vi "control.vi"() -> ()   [LabVIEW 2011]
uses:
  Controls/States.ctl
  <vilib>/Instr/_visa.llb/VISA Configure Serial Port (Instr).vi
panel:
  out "read buffer":string
  in  "Vertical Pointer Slide":dbl(slide) scale=0.0..100.0
  in  "Stop Button":bool
  in  "VISA resource name":refnum<visa-resource-name>
  in  "Stop Motion":bool caption="Stop"
  in  "Right":bool
  in  "Left":bool
  in  "Forward":bool
  in  "Back":bool
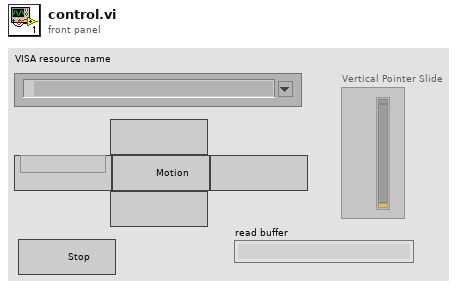
[diagram p1: front panel]
types:
  T1 = typedef "States.ctl" = enum16{"Init", "Idle", "AckCommand", "CheckError", "Shutdown"}
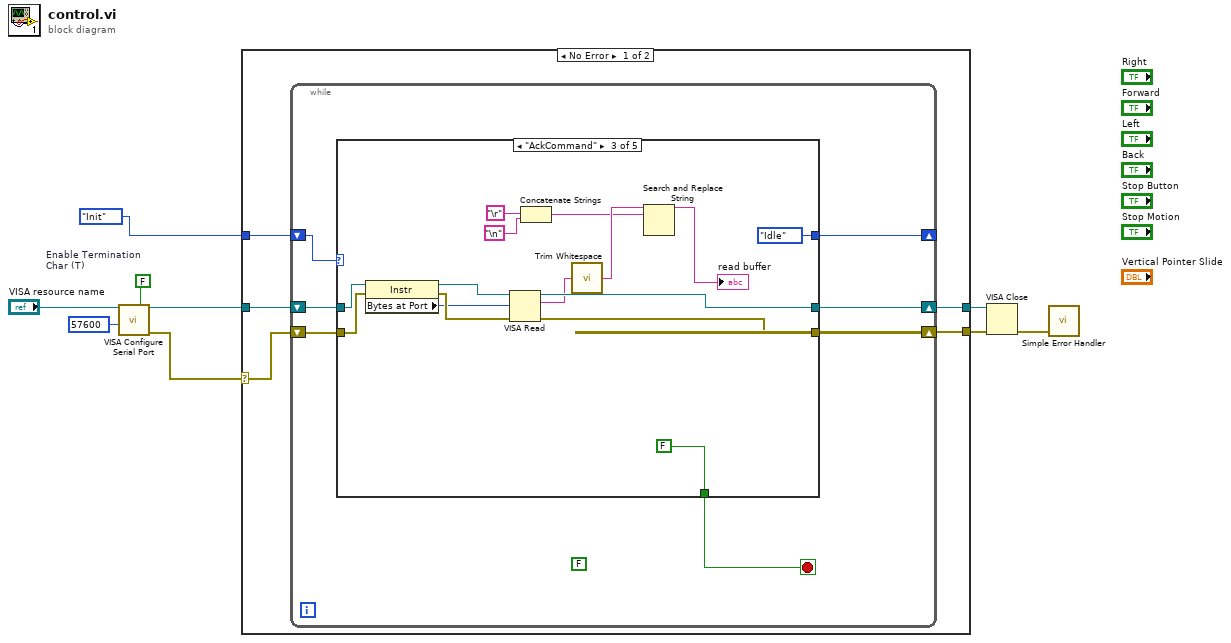
[diagram p0: block diagram]
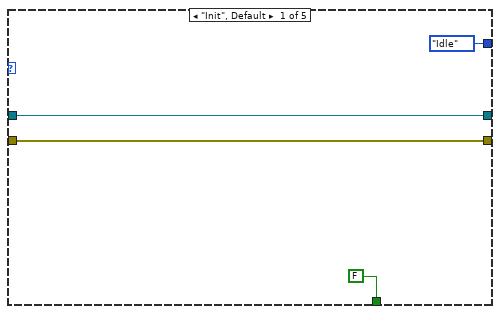
[diagram p2: hidden frame]
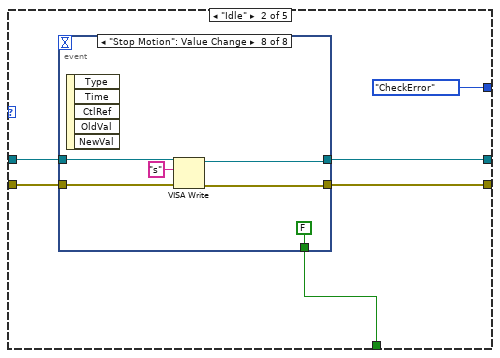
[diagram p3: hidden frame]
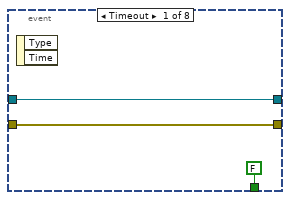
[diagram p4: hidden frame]
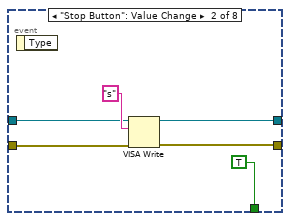
[diagram p5: hidden frame]
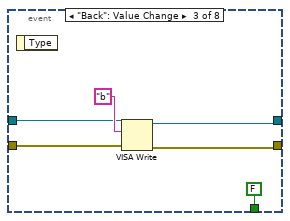
[diagram p6: hidden frame]
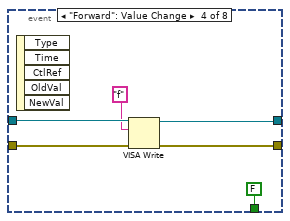
[diagram p7: hidden frame]
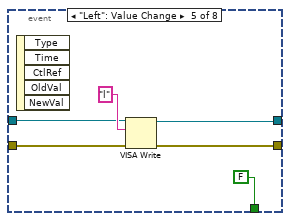
[diagram p8: hidden frame]
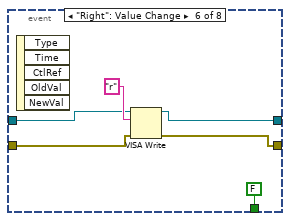
[diagram p9: hidden frame]
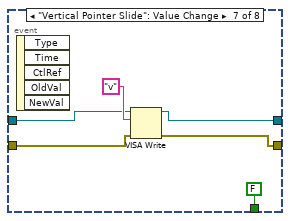
[diagram p10: hidden frame]
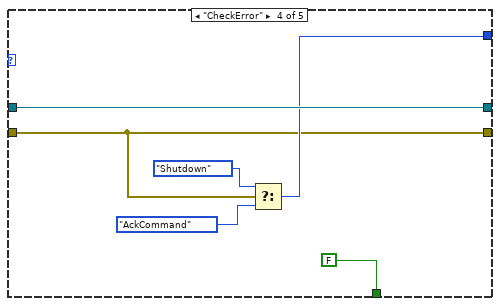
[diagram p11: hidden frame]
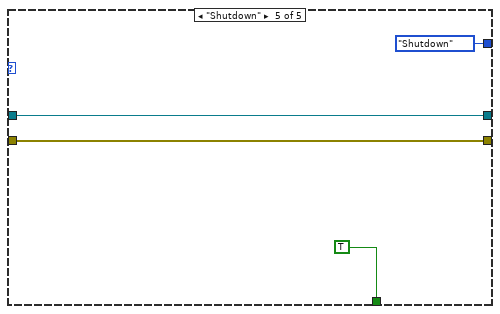
[diagram p12: hidden frame]
diagram:
  w1 = FALSE  # Enable Termination Char (T)
  n1 = call-poly "VISA Configure Serial Port"("VISA resource name"="VISA resource name", "Enable Termination\nChar (T)"=w1, "baud rate (9600)"=u32 57600) -> ("VISA resource name out"=w7:refnum<visa-resource-name>, "error out"=w2:errorcluster)  [unwired: 11 in]
  n2 = case shown="No Error" w2 {
    selector: w2 -> [w10 w102]
    tunnel: w7 -> [w14 w103]
    tunnel: [w13 w102] -> w6
    tunnel: [w12 w103] -> w5
    tunnel: States."Init" ("Enum") -> [w11 _]
    frame No Error {
      n3 = while {
        shift-right: [w15] -> _
        shift-left: w11 -> [w16]
        shift-right: [w17] -> w12
        shift-left: w14 -> [w18]
        shift-right: [w19] -> w13
        shift-left: w10 -> [w20]
        stop <- w21 stop-if-true
        (unwired) FALSE
        n4 = case shown="\"AckCommand\"" w16 {
          tunnel: [FALSE w31 FALSE FALSE TRUE] -> w21
          tunnel: w20 -> [w22 w30 w85 w93 w99]
          tunnel: [w22 w29 w83 w93 w99] -> w19
          tunnel: w18 -> [w23 w28 w86 w97 w100]
          tunnel: [w23 w27 w84 w97 w100] -> w17
          tunnel: [States."Idle" ("Enum") States."CheckError" ("Enum") States."Idle" ("Enum") w94 States."Shutdown" ("Enum")] -> w15
          frame "Init", Default {
          }
          frame "Idle" {
            n5 = event shown="[7] \"Stop Motion\": Value Change" {
              selector: _ -> [_ _ _ _ _ _ _ _]
              dyn-events: _ -> [_ _ _ _ _ _ _ _]
              timeout: _ -> [_ _ _ _ _ _ _ _]
              tunnel: [FALSE TRUE FALSE FALSE FALSE FALSE FALSE FALSE] -> w31
              tunnel: w30 -> [w32 w36 w43 w49 w55 w60 w66 w76]
              tunnel: [w32 w35 w42 w50 w54 w61 w67 w75] -> w29
              tunnel: w28 -> [w33 w38 w45 w52 w57 w63 w69 w74]
              tunnel: [w33 w37 w44 w51 w56 w62 w68 w73] -> w27
              event Timeout {
                n6 = event-data() -> ()  [unwired: 1 in, 2 out]
              }
              event "Stop Button": Value Change {
                n7 = event-data() -> ()  [unwired: 1 in, 1 out]
                n8 = VISA Write(VISA resource name=w38, write buffer="s", error in (no error)=w36) -> (VISA resource name out=w37:refnum<visa-resource-name>, error out=w35:errorcluster)  [unwired: 1 out]
              }
              event "Back": Value Change {
                n9 = event-data() -> ()  [unwired: 1 in, 1 out]
                n10 = VISA Write(VISA resource name=w45, write buffer="b", error in (no error)=w43) -> (VISA resource name out=w44:refnum<visa-resource-name>, error out=w42:errorcluster)  [unwired: 1 out]
              }
              event "Forward": Value Change {
                n11 = event-data() -> ()  [unwired: 1 in, 5 out]
                n12 = VISA Write(VISA resource name=w52, write buffer="f", error in (no error)=w49) -> (VISA resource name out=w51:refnum<visa-resource-name>, error out=w50:errorcluster)  [unwired: 1 out]
              }
              event "Left": Value Change {
                n13 = event-data() -> ()  [unwired: 1 in, 5 out]
                n14 = VISA Write(VISA resource name=w57, write buffer="l", error in (no error)=w55) -> (VISA resource name out=w56:refnum<visa-resource-name>, error out=w54:errorcluster)  [unwired: 1 out]
              }
              event "Right": Value Change {
                n15 = event-data() -> ()  [unwired: 1 in, 5 out]
                n16 = VISA Write(VISA resource name=w63, write buffer="r", error in (no error)=w60) -> (VISA resource name out=w62:refnum<visa-resource-name>, error out=w61:errorcluster)  [unwired: 1 out]
              }
              event "Vertical Pointer Slide": Value Change {
                n17 = event-data() -> ()  [unwired: 1 in, 5 out]
                n18 = VISA Write(VISA resource name=w69, write buffer="v", error in (no error)=w66) -> (VISA resource name out=w68:refnum<visa-resource-name>, error out=w67:errorcluster)  [unwired: 1 out]
              }
              event "Stop Motion": Value Change {
                n19 = event-data() -> ()  [unwired: 1 in, 5 out]
                n20 = VISA Write(VISA resource name=w74, write buffer="s", error in (no error)=w76) -> (VISA resource name out=w73:refnum<visa-resource-name>, error out=w75:errorcluster)  [unwired: 1 out]
              }
            }
          }
          frame "AckCommand" {
            n21 = property class="Instr"(reference=w86, error in=w85) -> (reference out=w89:refnum<visa-resource-name>, error out=w88:errorcluster, "Bytes at Port"=w87:u32)
            n22 = VISA Read(VISA resource name=w89, byte count=w87, error in (no error)=w88) -> (VISA resource name out=w84:refnum<visa-resource-name>, read buffer=w82:string, error out=w83:errorcluster)  [unwired: 1 out]
            n23 = Concatenate Strings("\r", "\n") -> (w78:string)
            n24 = call <vilib>:"Trim Whitespace.vi"("string"=w82) -> ("trimmed string"=w81:string)  [unwired: 1 in]
            n25 = Search and Replace String(input string=w81, search string=w78) -> (result string=→"read buffer":string)  [unwired: 6 in, 3 out]
          }
          frame "CheckError" {
            n26 = Select(t=States."Shutdown" ("Enum"), s=w93, f=States."AckCommand" ("Enum")) -> (s? t:f=w94:T1)
          }
          frame "Shutdown" {
          }
        }
      }
    }
    frame Error {
    }
  }
  n27 = VISA Close(VISA resource name=w5, error in (no error)=w6) -> (error out=w4:errorcluster)
  n28 = call <vilib>:"Simple Error Handler.vi"("error in (no error)"=w4) -> ()  [unwired: 4 in, 5 out]
